vi "Teleop.vi"(10 "Match Info":T3={"Autonomous Elapsed Seconds"=0.0, "TeleOp Elapsed Seconds"=0.0, "Disabled Elapsed Seconds"=0.0, "Visited Autonomous"=FALSE, "Visited TeleOp"=FALSE, "Visited Disabled"=FALSE, "Autonomous Settings"={"Autonomous Style"=enum."Independent", "VI Refnum"=refnum}}, 11 "Call Context":T4) -> ()   [LabVIEW 2011]
doc: "This VI is called for each TeleOp packet received from the DS where the robot is not disabled. It is often used to read from the joysticks and update I/O or to update setpoints for timed control loops. It should complete and return within 20 milliseconds or it may miss DS packets."
uses:
  <vilib>/Rock Robotics/WPI/DriverStation/WPI_DriverStationDerivedRobotMode.ctl
  <vilib>/Rock Robotics/WPI/DriverStation/WPI_DriverStationMatch Info.ctl
  <vilib>/Rock Robotics/WPI/Relay/WPI_RelayValue.ctl
  Robot Global Data.vi
  <vilib>/addons/control/pid/pid.llb/PID (DBL).vi
  <vilib>/addons/control/pid/NI_PID_pid.lvlib
panel:
  in  "PID gains":T1={"proportional gain (Kc)"=0.0006, "integral time (Ti, min)"=0.03333, "derivative time (Td, min)"=0.002} {"derivative time (Td, min)" format="%.5f"; "integral time (Ti, min)" format="%.5f"; "proportional gain (Kc)" format="%.5f"}
  in  "PID Setpoint":dbl(knob) scale=0.0..2000.0
  in  "Light":bool
  in  "Drive Mode":T2(ring)=enum."Manual"
  in  "RPM Set Point 2":dbl(knob) scale=0.0..2000.0
  in  "RPM Gain (Edan Test)":dbl
  in  "Right Wheel Gain":dbl
  in  "Left Wheel Gain":dbl
  out "pythagorean X":dbl(knob) scale=0.0..20.0
  out "camera distance":dbl(knob) scale=0.0..10.0
  out "Angle (X)":dbl
  out "pythagorean Y":dbl(knob) scale=0.0..20.0
  out "Angle (Y)":dbl
  in  "Boolean":bool
  in  "RPM Set Point":dbl(knob) scale=0.0..2000.0
  in  "Shooter Speed Gain":dbl=0.1
  in  "Angle Set Point":dbl(knob)=195.27022900531597 scale=180.0..220.0
  in  "Angle Gain":dbl
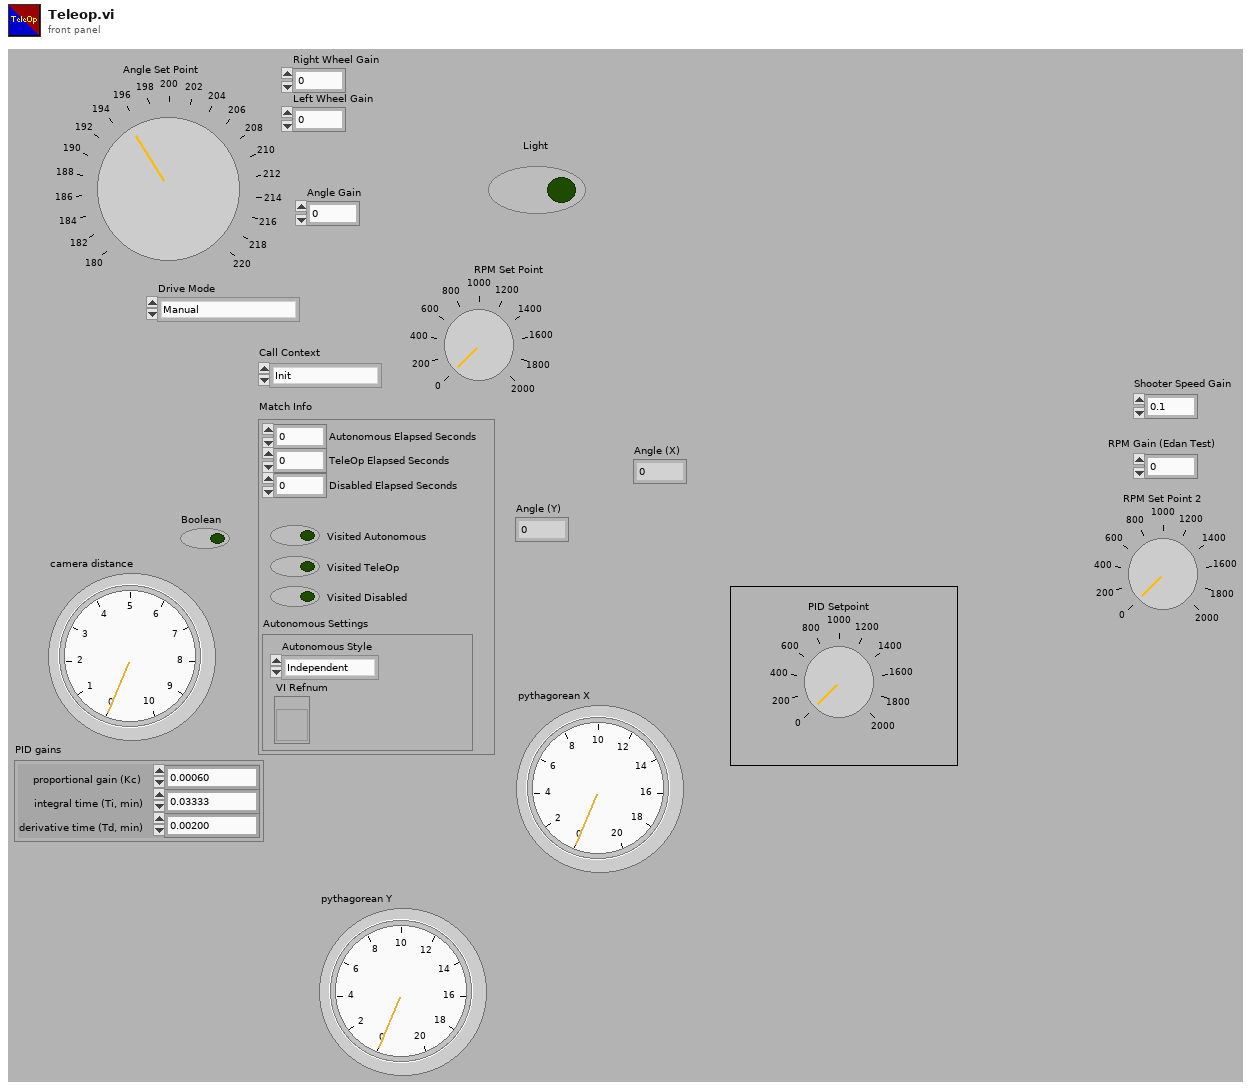
[diagram p1: front panel]
types:
  T1 = cluster{"proportional gain (Kc)":dbl, "integral time (Ti, min)":dbl, "derivative time (Td, min)":dbl}
  T2 = enum16{"Closed Loop Test", "PID Shooter Test", "camera", "ClosedLoopDrive", "Manual", "shooter test"}
  T3 = typedef "WPI_DriverStationMatch Info.ctl" = cluster{"Autonomous Elapsed Seconds":dbl, "TeleOp Elapsed Seconds":dbl, "Disabled Elapsed Seconds":dbl, "Visited Autonomous":bool, "Visited TeleOp":bool, "Visited Disabled":bool, "Autonomous Settings":cluster{"Autonomous Style":enum16{"Iterative", "Independent"}, "VI Refnum":refnum<vi>}}
  T4 = typedef "WPI_DriverStationDerivedRobotMode.ctl" = enum16{"Init", "Execute", "Stop"}
  T5 = typedef "WPI_RelayValue.ctl" = enum16{"Off", "On", "Forward", "Reverse"}
  T6 = typedef "WPI_MotorControlDeviceRef.ctl" = cluster{"DeviceStatus":errorcluster, "Type":enum16{"PWM", "CAN"}, "PWM":cluster{"Digital Module":T7, "PWM Channel":T8, "DeadBand":T9}, "CAN":cluster{"Device Number":u8, "Control Mode":T10, "Semaphore":T11, "Max Vout":dbl}, "Invert":bool, "TransformRef":T12, "InvTransformRef":T12}
  T7 = typedef "FPGA_TypedefDigitalModule.ctl" = enum16{"Digital Module 1", "Digital Module 2"}
  T8 = typedef "FPGA_DIOPWMChannel.ctl" = enum8{"PWM 1", "PWM 2", "PWM 3", "PWM 4", "PWM 5", "PWM 6", "PWM 7", "PWM 8", "PWM 9", "PWM 10", "Invalid"}
  T9 = typedef "WPI_PWMDeadband.ctl" = cluster{"Name":string, "maxPositivePwm":i32, "minPositivePwm":i32, "centerPwm":i32, "maxNegativePwm":i32, "minNegativePwm":i32, "angularRange":u16}
  T10 = typedef "WPI_CANJaguar_ControlMode.ctl" = enum8{"Percent VBus", "Current", "Speed", "Position", "Voltage"}
  T11 = typedef "Semaphore RefNum" = refnum<k1>
  T12 = typedef "WPI_PWMTransform_ConPane.ctl" = refnum<vi>
  T13 = typedef "WPI_DigitalInputDevRef.ctl" = cluster{"DevStatus":errorcluster, "DIO Channel":T14, "Digital Module":T7}
  T14 = typedef "FPGA_DIOChannel.ctl" = enum8{"DIO 1", "DIO 2", "DIO 3", "DIO 4", "DIO 5", "DIO 6", "DIO 7", "DIO 8", "DIO 9", "DIO 10", "DIO 11", "DIO 12", "DIO 13", "DIO 14", "Invalid"}
  T15 = typedef "WPI_JoystickDevRef.ctl" = cluster{"Device":T16}
  T16 = typedef "WPI_JoystickDeviceEnum.ctl" = enum16{"USB 1", "USB 2", "USB 3", "USB 4", "Kinect 1", "Kinect 2"}
  T17 = typedef "WPI_JoystickButtonState.ctl" = cluster{"Button 1":bool, "Button 2":bool, "Button 3":bool, "Button 4":bool, "Button 5":bool, "Button 6":bool, "Button 7":bool, "Button 8":bool, "Button 9":bool, "Button 10":bool, "Button 11":bool, "Button 12":bool}
  T18 = cluster{"axis 1 (x)":dbl, "axis 2 (y)":dbl, "axis 3 (throttle)":dbl, "axis 4":dbl, "axis 5":dbl, "axis 6":dbl}
  T19 = typedef "WPI_RelayDevRef.ctl" = cluster{"DevStatus":errorcluster, "Relay Channel":T20, "Digital Module":T7, "Relay Direction":T21}
  T20 = typedef "FPGA_DIORelayChannel.ctl" = enum8{"Relay 1", "Relay 2", "Relay 3", "Relay 4", "Relay 5", "Relay 6", "Relay 7", "Relay 8", "Invalid"}
  T21 = typedef "WPI_RelayDirection.ctl" = enum16{"Both directions", "Forward only", "Reverse only"}
  T22 = typedef "WPI_RobotDriveDevRef.ctl" = cluster{"DevStatus":errorcluster, "Motors[]":T6[], "Square Inputs":bool, "Max Output":dbl, "Isochronous":bool}
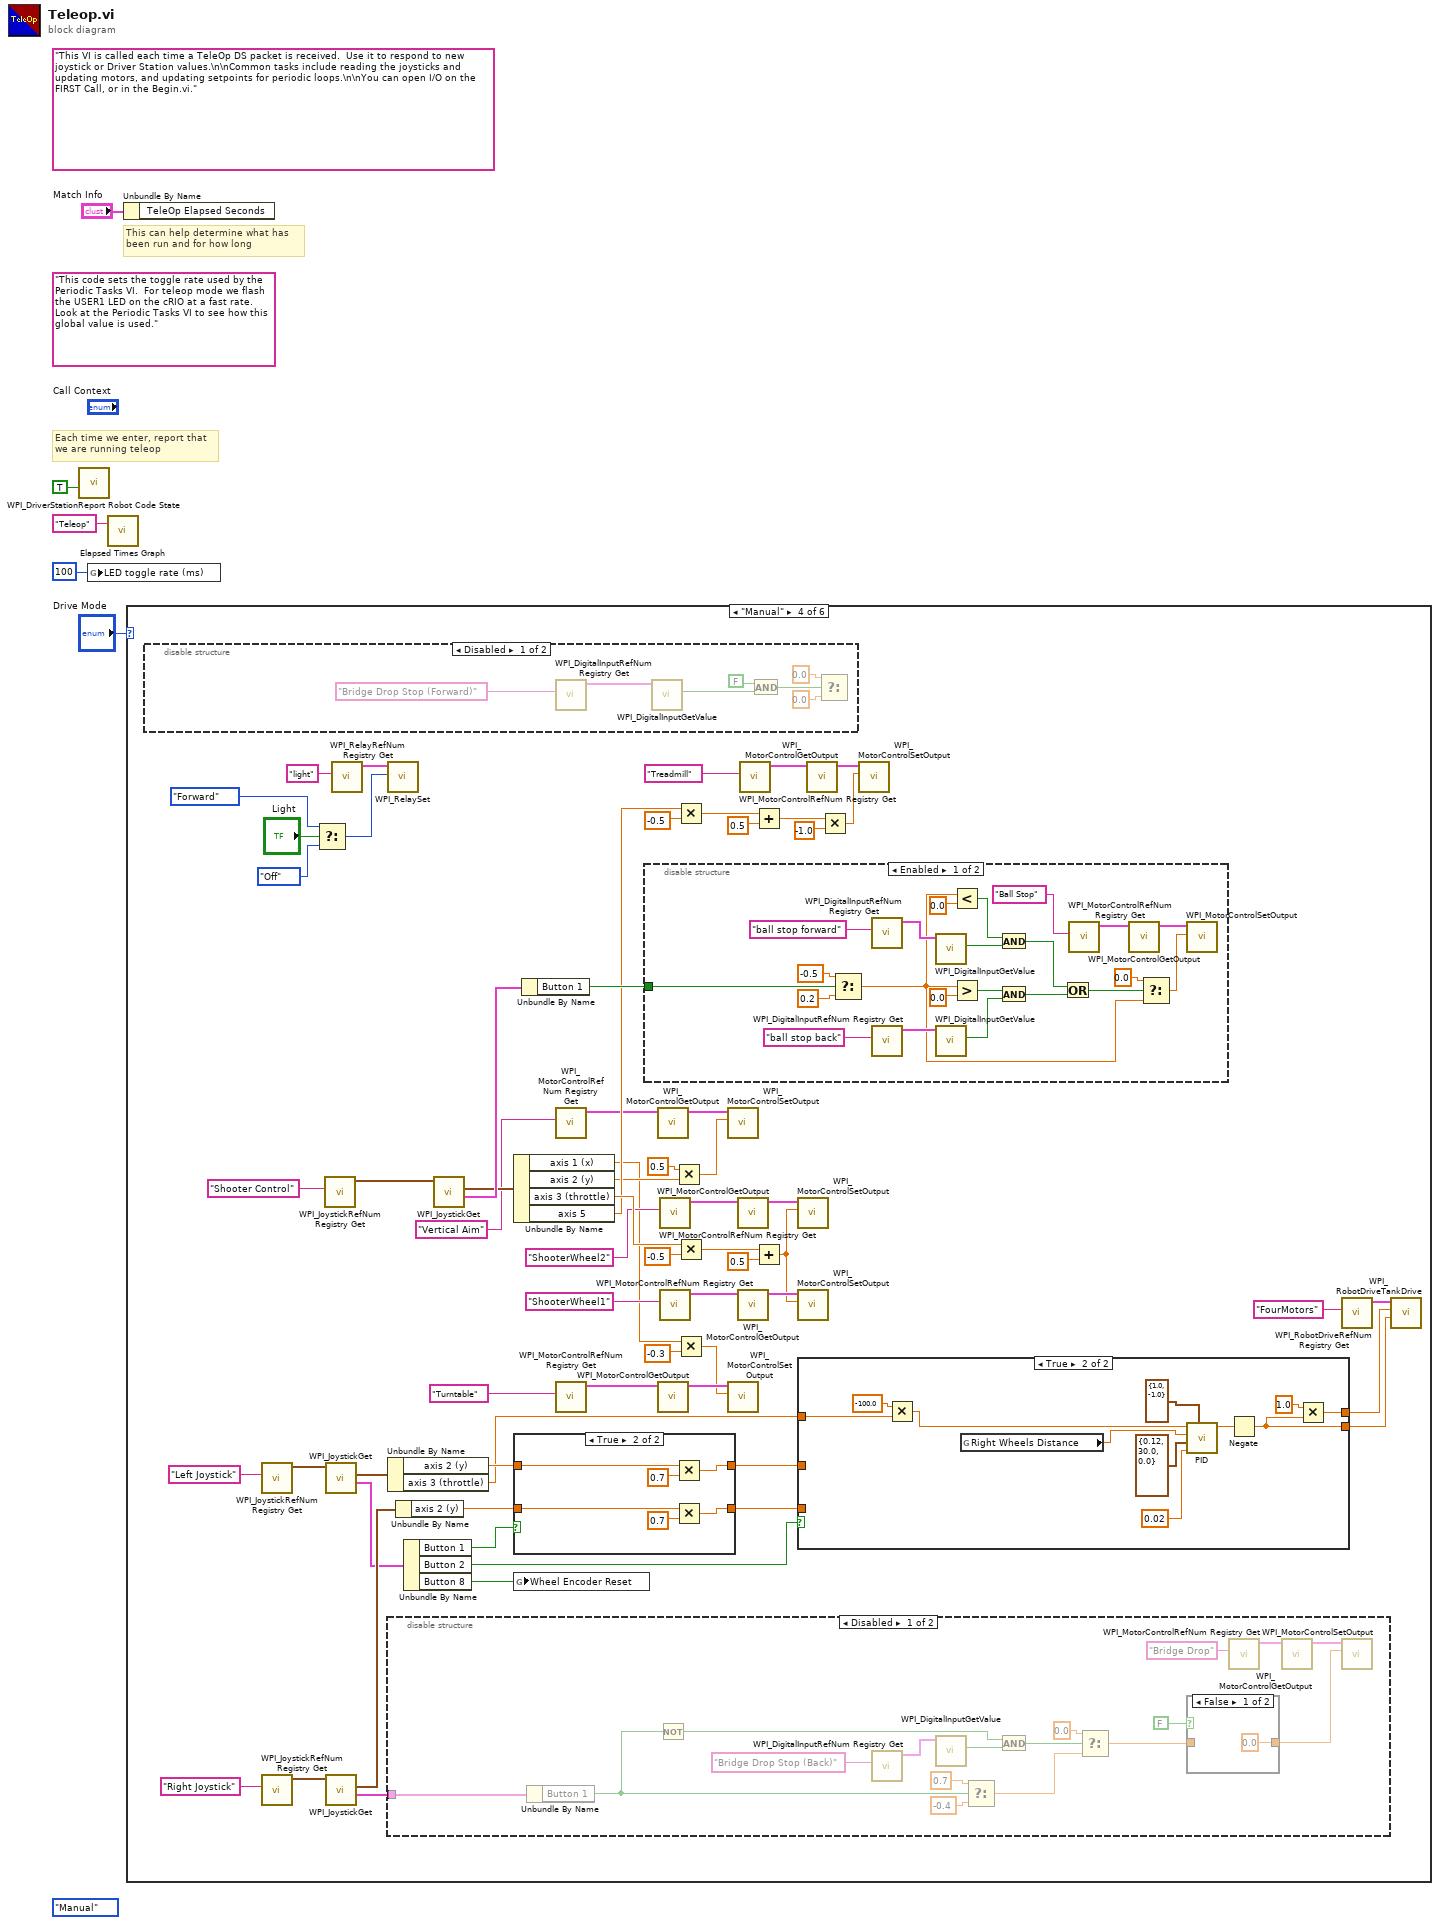
[diagram p0: block diagram]
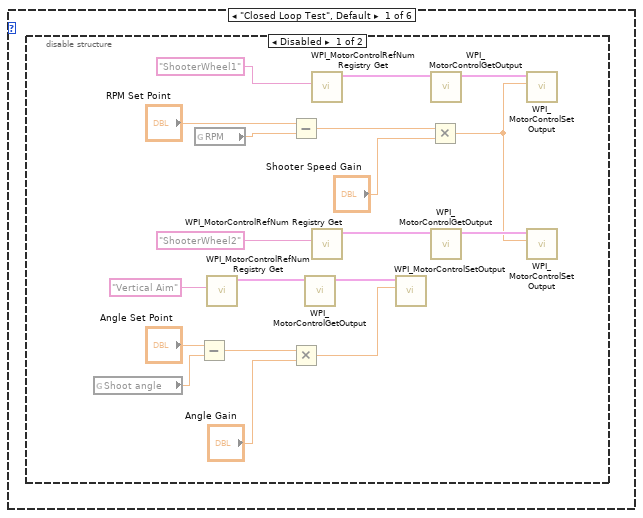
[diagram p2: hidden frame]
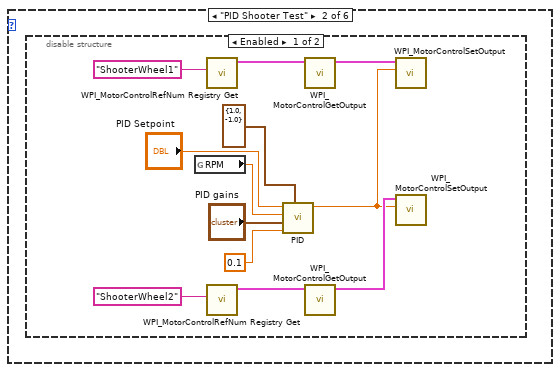
[diagram p4: hidden frame]
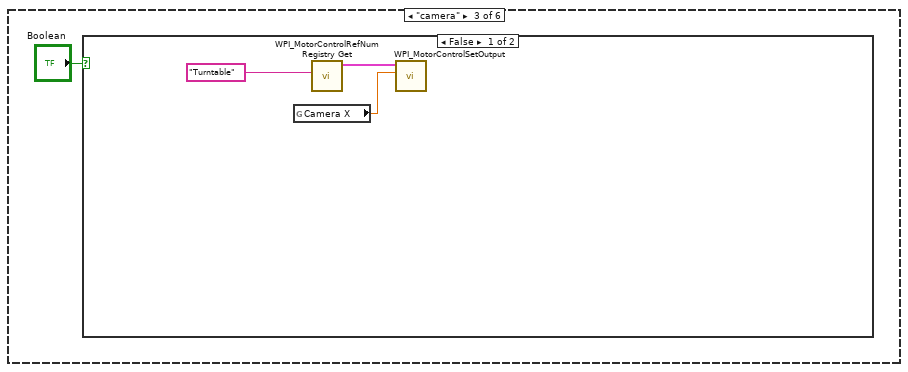
[diagram p6: hidden frame]
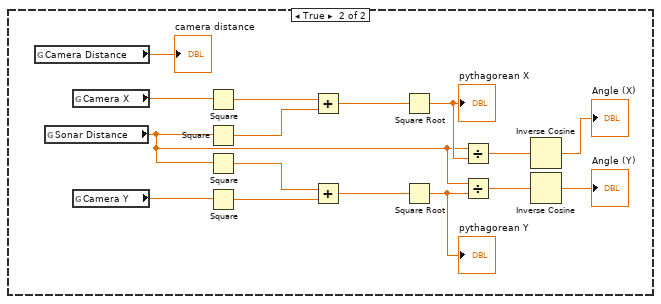
[diagram p7: hidden frame]
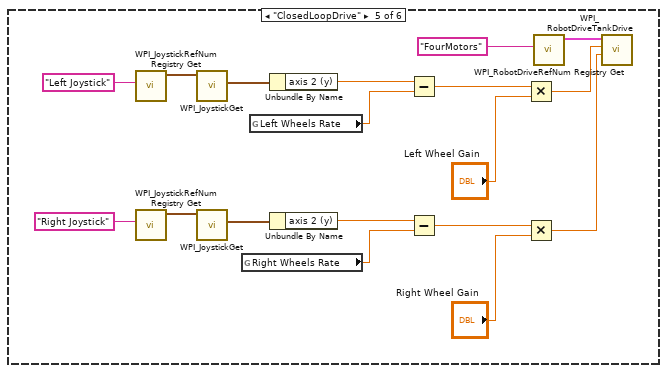
[diagram p14: hidden frame]
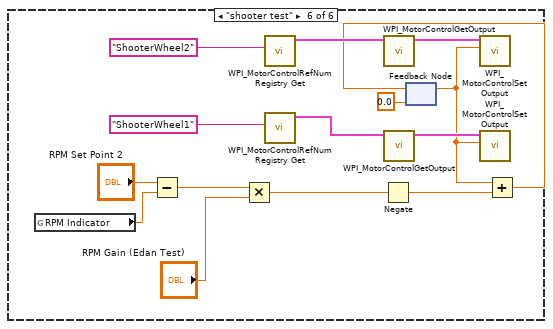
[diagram p15: hidden frame]
diagram:
  (unwired) T2."Manual" ("Drive Mode")
  (unwired) "This code sets the toggle rate used by the Periodic Tasks VI.  For teleop mode we flash the USER1 LED on the cRIO at a fast rate.  Look at the Periodic Tasks VI to see how this global value is used."
  (unwired) "This VI is called each time a TeleOp DS packet is received.  Use it to respond to new joystick or Driver Station values.\n\nCommon tasks include reading the joysticks and updating motors, and updating setpoints for periodic loops.\n\nYou can open I/O on the FIRST Call, or in the Begin.vi."
  # "Each time we enter, report that\nwe are running teleop"
  # "This can help determine what has\nbeen run and for how long"
  n1 = call <vilib>:"WPI_DriverStationReport Robot Code State.vi"("TeleOp"=TRUE ("Autonomous")) -> ()  [unwired: 10 in, 1 out]
  n2 = global write "Robot Global Data.vi" "LED toggle rate (ms)"(u32 100 ("LED ms toggle rate")) -> ()
  n3 = call "Elapsed Times Graph.vi"("User Identification:"="Teleop") -> ()  [unwired: 3 in]
  n4 = Unbundle By Name("Match Info") -> ()  [unwired: 1 out]
  n5 = case shown="\"Manual\"" "Drive Mode" {
    frame "Closed Loop Test", Default {
      n6 = disable-structure shown="Disabled" {
        frame Disabled {
          n7 = global read "Robot Global Data.vi" "Shoot angle"() -> (w14:dbl)
          n8 = global read "Robot Global Data.vi" "RPM"() -> (w18:dbl)
          n9 = Subtract(x="Angle Set Point", y=w14) -> (x-y=w12:dbl)
          n10 = call <vilib>:"WPI_MotorControlRefNum Registry Get.vi"("refnum name"="Vertical Aim") -> ("MotorControlDevRef"=w8:T6)  [unwired: 9 in, 1 out]
          n11 = Subtract(x="RPM Set Point", y=w18) -> (x-y=w16:dbl)
          n12 = Multiply(x=w12, y="Angle Gain") -> (x*y=w10:dbl)
          n13 = call <vilib>:"WPI_MotorControlGetOutput.vi"("MotorControlDevRef"=w8) -> ("MotorControlDevRef"=w9:T6)  [unwired: 8 in, 2 out]
          n14 = call <vilib>:"WPI_MotorControlRefNum Registry Get.vi"("refnum name"="ShooterWheel1") -> ("MotorControlDevRef"=w19:T6)  [unwired: 9 in, 1 out]
          n15 = call <vilib>:"WPI_MotorControlRefNum Registry Get.vi"("refnum name"="ShooterWheel2") -> ("MotorControlDevRef"=w23:T6)  [unwired: 9 in, 1 out]
          n16 = call <vilib>:"WPI_MotorControlSetOutput.vi"("Output"=w10, "MotorControlDevRef"=w9) -> ()  [unwired: 8 in, 2 out]
          n17 = Multiply(x=w16, y="Shooter Speed Gain") -> (x*y=w6:dbl)
          n18 = call <vilib>:"WPI_MotorControlGetOutput.vi"("MotorControlDevRef"=w19) -> ("MotorControlDevRef"=w20:T6)  [unwired: 8 in, 2 out]
          n19 = call <vilib>:"WPI_MotorControlGetOutput.vi"("MotorControlDevRef"=w23) -> ("MotorControlDevRef"=w22:T6)  [unwired: 8 in, 2 out]
          n20 = call <vilib>:"WPI_MotorControlSetOutput.vi"("Output"=w6, "MotorControlDevRef"=w20) -> ()  [unwired: 8 in, 2 out]
          n21 = call <vilib>:"WPI_MotorControlSetOutput.vi"("Output"=w6, "MotorControlDevRef"=w22) -> ()  [unwired: 8 in, 2 out]
        }
        frame Enabled {
        }
      }
    }
    frame "PID Shooter Test" {
      n22 = disable-structure shown="Enabled" {
        frame Enabled {
          n23 = global read "Robot Global Data.vi" "RPM"() -> (w30:dbl)
          n24 = call <vilib>:"WPI_MotorControlRefNum Registry Get.vi"("refnum name"="ShooterWheel1") -> ("MotorControlDevRef"=w31:T6)  [unwired: 9 in, 1 out]
          n25 = call <vilib>:"WPI_MotorControlRefNum Registry Get.vi"("refnum name"="ShooterWheel2") -> ("MotorControlDevRef"=w35:T6)  [unwired: 9 in, 1 out]
          n26 = call-poly <vilib>:"PID.vi"("output range"=cluster{"output high":dbl, "output low":dbl} {"output high"=1.0, "output low"=-1.0}, "dt (s)"=0.1, "PID gains"="PID gains", "process variable"=w30, "setpoint"="PID Setpoint") -> ("output"=w26:dbl)  [unwired: 5 in, 1 out]
          n27 = call <vilib>:"WPI_MotorControlGetOutput.vi"("MotorControlDevRef"=w31) -> ("MotorControlDevRef"=w32:T6)  [unwired: 8 in, 2 out]
          n28 = call <vilib>:"WPI_MotorControlGetOutput.vi"("MotorControlDevRef"=w35) -> ("MotorControlDevRef"=w34:T6)  [unwired: 8 in, 2 out]
          n29 = call <vilib>:"WPI_MotorControlSetOutput.vi"("Output"=w26, "MotorControlDevRef"=w32) -> ()  [unwired: 8 in, 2 out]
          n30 = call <vilib>:"WPI_MotorControlSetOutput.vi"("Output"=w26, "MotorControlDevRef"=w34) -> ()  [unwired: 8 in, 2 out]
        }
        frame Disabled {
        }
      }
    }
    frame "camera" {
      n31 = case shown="False" "Boolean" {
        frame False {
          n32 = global read "Robot Global Data.vi" "Camera X"() -> (w38:dbl)
          n33 = call <vilib>:"WPI_MotorControlRefNum Registry Get.vi"("refnum name"="Turntable") -> ("MotorControlDevRef"=w40:T6)  [unwired: 9 in, 1 out]
          n34 = call <vilib>:"WPI_MotorControlSetOutput.vi"("Output"=w38, "MotorControlDevRef"=w40) -> ()  [unwired: 8 in, 2 out]
        }
        frame True {
          n35 = global read "Robot Global Data.vi" "Camera Distance"() -> (→"camera distance":dbl)
          n36 = global read "Robot Global Data.vi" "Sonar Distance"() -> (w53:dbl)
          n37 = global read "Robot Global Data.vi" "Camera X"() -> (w55:dbl)
          n38 = global read "Robot Global Data.vi" "Camera Y"() -> (w49:dbl)
          n39 = Square(x=w55) -> (x^2=w42:dbl)
          n40 = Square(x=w53) -> (x^2=w41:dbl)
          n41 = Square(x=w53) -> (x^2=w46:dbl)
          n42 = Square(x=w49) -> (x^2=w47:dbl)
          n43 = Add(x=w42, y=w41) -> (x+y=w43:dbl)
          n44 = Add(x=w46, y=w47) -> (x+y=w48:dbl)
          n45 = Square Root(x=w43) -> (sqrt(x)=w54:dbl)
          "pythagorean X" <- w54
          n46 = Square Root(x=w48) -> (sqrt(x)=w52:dbl)
          "pythagorean Y" <- w52
          n47 = Divide(x=w53, y=w54) -> (x/y=w45:dbl)
          n48 = Divide(x=w53, y=w52) -> (x/y=w50:dbl)
          n49 = Inverse Cosine(1:w45) -> (0:→"Angle (X)":dbl)
          n50 = Inverse Cosine(1:w50) -> (0:→"Angle (Y)":dbl)
        }
      }
    }
    frame "Manual" {
      n51 = disable-structure shown="Disabled" {
        frame Disabled {
          n52 = call <vilib>:"WPI_DigitalInputRefNum Registry Get.vi"("refnum name"="Bridge Drop Stop (Forward)") -> ("DigitalInputDevRef"=w159:T13)  [unwired: 9 in, 1 out]
          n53 = call <vilib>:"WPI_DigitalInputGetValue.vi"("DigitalInputDevRef"=w159) -> ("Value"=w158:bool)  [unwired: 8 in, 2 out]
          n54 = And(x=FALSE, y=w158) -> (x .and. y?=w157:bool)
          n55 = Select(t=0.0, s=w157, f=0.0) -> ()  [unwired: 1 out]
        }
        frame Enabled {
        }
      }
      n56 = call <vilib>:"WPI_JoystickRefNum Registry Get.vi"("refnum name"="Left Joystick") -> ("JoystickDevRef"=w115:T15)  [unwired: 9 in, 1 out]
      n57 = call <vilib>:"WPI_JoystickRefNum Registry Get.vi"("refnum name"="Right Joystick") -> ("JoystickDevRef"=w118:T15)  [unwired: 9 in, 1 out]
      n58 = Select(t=WPI_RelayValue."Forward" ("RelayValue"), s="Light", f=WPI_RelayValue."Off" ("RelayValue")) -> (s? t:f=w71:T5)
      n59 = call <vilib>:"WPI_JoystickRefNum Registry Get.vi"("refnum name"="Shooter Control") -> ("JoystickDevRef"=w88:T15)  [unwired: 9 in, 1 out]
      n60 = call <vilib>:"WPI_JoystickGet.vi"("JoystickDevRef"=w115) -> ("Buttons"=w67:T17, "Axes"=w116:T18)  [unwired: 4 in, 1 out]
      n61 = call <vilib>:"WPI_JoystickGet.vi"("JoystickDevRef"=w118) -> ("Buttons"=w77:T17, "Axes"=w119:T18)  [unwired: 4 in, 1 out]
      n62 = call <vilib>:"WPI_RelayRefNum Registry Get.vi"("refnum name"="light") -> ("RelayDevRef"=w75:T19)  [unwired: 9 in, 1 out]
      n63 = call <vilib>:"WPI_RelaySet.vi"("RelayValue"=w71, "RelayDevRef"=w75) -> ()  [unwired: 8 in, 2 out]
      n64 = Unbundle By Name(w116) -> ("axis 2 (y)"=w69:dbl, "axis 3 (throttle)"=w58:dbl)
      n65 = disable-structure shown="Disabled" {
        disable-tunnel: w77 -> [w150 _]
        frame Disabled {
          n66 = Unbundle By Name(w150) -> ("Button 1"=w144:bool)
          n67 = Not(x=w144) -> (.not. x?=w145:bool)
          n68 = call <vilib>:"WPI_DigitalInputRefNum Registry Get.vi"("refnum name"="Bridge Drop Stop (Back)") -> ("DigitalInputDevRef"=w147:T13)  [unwired: 9 in, 1 out]
          n69 = call <vilib>:"WPI_DigitalInputGetValue.vi"("DigitalInputDevRef"=w147) -> ("Value"=w140:bool)  [unwired: 8 in, 2 out]
          n70 = Select(t=0.7, s=w144, f=-0.4) -> (s? t:f=w139:dbl)
          n71 = And(x=w145, y=w140) -> (x .and. y?=w146:bool)
          n72 = Select(t=0.0, s=w146, f=w139) -> (s? t:f=w141:dbl)
          n73 = case shown="False" FALSE {
            tunnel: [0.0 ("f") w152] -> w134
            tunnel: w141 -> [_ w152]
            frame False {
            }
            frame True {
            }
          }
          n74 = call <vilib>:"WPI_MotorControlRefNum Registry Get.vi"("refnum name"="Bridge Drop") -> ("MotorControlDevRef"=w138:T6)  [unwired: 9 in, 1 out]
          n75 = call <vilib>:"WPI_MotorControlGetOutput.vi"("MotorControlDevRef"=w138) -> ("MotorControlDevRef"=w137:T6)  [unwired: 8 in, 2 out]
          n76 = call <vilib>:"WPI_MotorControlSetOutput.vi"("Output"=w134, "MotorControlDevRef"=w137) -> ()  [unwired: 8 in, 2 out]
        }
        frame Enabled {
        }
      }
      n77 = Unbundle By Name(w119) -> ("axis 2 (y)"=w68:dbl)
      n78 = Unbundle By Name(w67) -> ("Button 1"=w66:bool, "Button 2"=w60:bool, "Button 8"=w57:bool)
      n79 = call <vilib>:"WPI_JoystickGet.vi"("JoystickDevRef"=w88) -> ("Buttons"=w111:T17, "Axes"=w90:T18)  [unwired: 4 in, 1 out]
      n80 = Unbundle By Name(w90) -> ("axis 1 (x)"=w78:dbl, "axis 2 (y)"=w83:dbl, "axis 3 (throttle)"=w110:dbl, "axis 5"=w109:dbl)
      n81 = case shown="True" w66 {
        tunnel: [w161 w167] -> w63
        tunnel: w69 -> [w161 w164]
        tunnel: [w160 w166] -> w61
        tunnel: w68 -> [w160 w165]
        frame False {
        }
        frame True {
          n82 = Multiply(x=w164, y=0.7) -> (x*y=w167:dbl)
          n83 = Multiply(x=w165, y=0.7) -> (x*y=w166:dbl)
        }
      }
      n84 = global write "Robot Global Data.vi" "Wheel Encoder Reset"(w57) -> ()
      n85 = Unbundle By Name(w111) -> ("Button 1"=w112:bool)
      n86 = call <vilib>:"WPI_MotorControlRefNum Registry Get.vi"("refnum name"="Vertical Aim") -> ("MotorControlDevRef"=w86:T6)  [unwired: 9 in, 1 out]
      n87 = call <vilib>:"WPI_MotorControlRefNum Registry Get.vi"("refnum name"="Turntable") -> ("MotorControlDevRef"=w107:T6)  [unwired: 9 in, 1 out]
      n88 = disable-structure shown="Enabled" {
        disable-tunnel: w112 -> [w187 _]
        frame Enabled {
          n89 = Select(t=-0.5, s=w187, f=0.2) -> (s? t:f=w174:dbl)
          n90 = call <vilib>:"WPI_DigitalInputRefNum Registry Get.vi"("refnum name"="ball stop forward") -> ("DigitalInputDevRef"=w180:T13)  [unwired: 9 in, 1 out]
          n91 = call <vilib>:"WPI_DigitalInputRefNum Registry Get.vi"("refnum name"="ball stop back") -> ("DigitalInputDevRef"=w179:T13)  [unwired: 9 in, 1 out]
          n92 = call <vilib>:"WPI_DigitalInputGetValue.vi"("DigitalInputDevRef"=w180) -> ("Value"=w169:bool)  [unwired: 8 in, 2 out]
          n93 = call <vilib>:"WPI_DigitalInputGetValue.vi"("DigitalInputDevRef"=w179) -> ("Value"=w168:bool)  [unwired: 8 in, 2 out]
          n94 = Less?(x=w174, y=0.0) -> (x < y?=w170:bool)
          n95 = Greater?(x=w174, y=0.0) -> (0:w171:bool)
          n96 = And(x=w170, y=w169) -> (x .and. y?=w183:bool)
          n97 = And(x=w171, y=w168) -> (x .and. y?=w182:bool)
          n98 = Or(x=w183, y=w182) -> (x .or. y?=w181:bool)
          n99 = call <vilib>:"WPI_MotorControlRefNum Registry Get.vi"("refnum name"="Ball Stop") -> ("MotorControlDevRef"=w172:T6)  [unwired: 9 in, 1 out]
          n100 = call <vilib>:"WPI_MotorControlGetOutput.vi"("MotorControlDevRef"=w172) -> ("MotorControlDevRef"=w176:T6)  [unwired: 8 in, 2 out]
          n101 = Select(t=0.0, s=w181, f=w174) -> (s? t:f=w175:dbl)
          n102 = call <vilib>:"WPI_MotorControlSetOutput.vi"("Output"=w175, "MotorControlDevRef"=w176) -> ()  [unwired: 8 in, 2 out]
        }
        frame Disabled {
        }
      }
      n103 = call <vilib>:"WPI_MotorControlGetOutput.vi"("MotorControlDevRef"=w86) -> ("MotorControlDevRef"=w82:T6)  [unwired: 8 in, 2 out]
      n104 = call <vilib>:"WPI_MotorControlGetOutput.vi"("MotorControlDevRef"=w107) -> ("MotorControlDevRef"=w106:T6)  [unwired: 8 in, 2 out]
      n105 = call <vilib>:"WPI_MotorControlRefNum Registry Get.vi"("refnum name"="ShooterWheel2") -> ("MotorControlDevRef"=w101:T6)  [unwired: 9 in, 1 out]
      n106 = call <vilib>:"WPI_MotorControlRefNum Registry Get.vi"("refnum name"="ShooterWheel1") -> ("MotorControlDevRef"=w97:T6)  [unwired: 9 in, 1 out]
      n107 = Multiply(x=0.5 ("y"), y=w83) -> (x*y=w84:dbl)
      n108 = Multiply(x=w109, y=-0.5) -> (x*y=w94:dbl)
      n109 = Multiply(x=w110, y=-0.5) -> (x*y=w104:dbl)
      n110 = Multiply(x=w78, y=-0.3) -> (x*y=w65:dbl)
      n111 = call <vilib>:"WPI_MotorControlSetOutput.vi"("Output"=w84, "MotorControlDevRef"=w82) -> ()  [unwired: 8 in, 2 out]
      n112 = call <vilib>:"WPI_MotorControlSetOutput.vi"("Output"=w65, "MotorControlDevRef"=w106) -> ()  [unwired: 8 in, 2 out]
      n113 = call <vilib>:"WPI_MotorControlGetOutput.vi"("MotorControlDevRef"=w101) -> ("MotorControlDevRef"=w100:T6)  [unwired: 8 in, 2 out]
      n114 = call <vilib>:"WPI_MotorControlGetOutput.vi"("MotorControlDevRef"=w97) -> ("MotorControlDevRef"=w98:T6)  [unwired: 8 in, 2 out]
      n115 = call <vilib>:"WPI_MotorControlRefNum Registry Get.vi"("refnum name"="Treadmill") -> ("MotorControlDevRef"=w92:T6)  [unwired: 9 in, 1 out]
      n116 = Add(x=w94, y=0.5) -> (x+y=w79:dbl)
      n117 = Add(x=w104, y=0.5) -> (x+y=w76:dbl)
      n118 = call <vilib>:"WPI_MotorControlSetOutput.vi"("Output"=w76, "MotorControlDevRef"=w100) -> ()  [unwired: 8 in, 2 out]
      n119 = call <vilib>:"WPI_MotorControlSetOutput.vi"("Output"=w76, "MotorControlDevRef"=w98) -> ()  [unwired: 8 in, 2 out]
      n120 = case shown="True" w60 {
        tunnel: [w122 w125] -> w59
        tunnel: w63 -> [w122 _]
        tunnel: [w121 w124] -> w62
        tunnel: w61 -> [w121 _]
        tunnel: w58 -> [_ w132]
        frame False {
        }
        frame True {
          n121 = Multiply(x=-100.0, y=w132) -> (x*y=w133:dbl)
          n122 = global read "Robot Global Data.vi" "Right Wheels Distance"() -> (w130:dbl)
          n123 = call-poly <vilib>:"PID.vi"("output range"=cluster{"output high":dbl, "output low":dbl} {"output high"=1.0, "output low"=-1.0}, "dt (s)"=0.02, "PID gains"=T1 {"proportional gain (Kc)"=0.12, "integral time (Ti, min)"=30.0, "derivative time (Td, min)"=0.0}, "process variable"=w130, "setpoint"=w133) -> ("output"=w126:dbl)  [unwired: 5 in, 1 out]
          n124 = Negate(x=w126) -> (-x=w124:dbl)
          n125 = Multiply(x=1.0, y=w124) -> (x*y=w125:dbl)
        }
      }
      n126 = call <vilib>:"WPI_MotorControlGetOutput.vi"("MotorControlDevRef"=w92) -> ("MotorControlDevRef"=w91:T6)  [unwired: 8 in, 2 out]
      n127 = Multiply(x=w79, y=-1.0) -> (x*y=w80:dbl)
      n128 = call <vilib>:"WPI_MotorControlSetOutput.vi"("Output"=w80, "MotorControlDevRef"=w91) -> ()  [unwired: 8 in, 2 out]
      n129 = call <vilib>:"WPI_RobotDriveRefNum Registry Get.vi"("refnum name"="FourMotors") -> ("RobotDriveDevRef"=w114:T22)  [unwired: 1 in, 9 out]
      n130 = call <vilib>:"WPI_RobotDriveTankDrive.vi"("Right axis value"=w62, "Left axis value"=w59, "RobotDriveDevRef"=w114) -> ()  [unwired: 7 in, 2 out]
    }
    frame "ClosedLoopDrive" {
      n131 = call <vilib>:"WPI_JoystickRefNum Registry Get.vi"("refnum name"="Left Joystick") -> ("JoystickDevRef"=w202:T15)  [unwired: 9 in, 1 out]
      n132 = call <vilib>:"WPI_JoystickRefNum Registry Get.vi"("refnum name"="Right Joystick") -> ("JoystickDevRef"=w205:T15)  [unwired: 9 in, 1 out]
      n133 = call <vilib>:"WPI_JoystickGet.vi"("JoystickDevRef"=w202) -> ("Axes"=w203:T18)  [unwired: 4 in, 2 out]
      n134 = call <vilib>:"WPI_JoystickGet.vi"("JoystickDevRef"=w205) -> ("Axes"=w206:T18)  [unwired: 4 in, 2 out]
      n135 = global read "Robot Global Data.vi" "Right Wheels Rate"() -> (w198:dbl)
      n136 = global read "Robot Global Data.vi" "Left Wheels Rate"() -> (w196:dbl)
      n137 = Unbundle By Name(w203) -> ("axis 2 (y)"=w197:dbl)
      n138 = Unbundle By Name(w206) -> ("axis 2 (y)"=w199:dbl)
      n139 = Subtract(x=w197, y=w196) -> (x-y=w195:dbl)
      n140 = Subtract(x=w199, y=w198) -> (x-y=w193:dbl)
      n141 = Multiply(x=w195, y="Left Wheel Gain") -> (x*y=w194:dbl)
      n142 = Multiply(x=w193, y="Right Wheel Gain") -> (x*y=w192:dbl)
      n143 = call <vilib>:"WPI_RobotDriveRefNum Registry Get.vi"("refnum name"="FourMotors") -> ("RobotDriveDevRef"=w201:T22)  [unwired: 1 in, 9 out]
      n144 = call <vilib>:"WPI_RobotDriveTankDrive.vi"("Right axis value"=w192, "Left axis value"=w194, "RobotDriveDevRef"=w201) -> ()  [unwired: 7 in, 2 out]
    }
    frame "shooter test" {
      n145 = global read "Robot Global Data.vi" "RPM Indicator"() -> (w220:dbl)
      n146 = Subtract(x="RPM Set Point 2", y=w220) -> (x-y=w222:dbl)
      n147 = Multiply(x=w222, y="RPM Gain (Edan Test)") -> (x*y=w213:dbl)
      n148 = call <vilib>:"WPI_MotorControlRefNum Registry Get.vi"("refnum name"="ShooterWheel2") -> ("MotorControlDevRef"=w215:T6)  [unwired: 9 in, 1 out]
      n149 = call <vilib>:"WPI_MotorControlRefNum Registry Get.vi"("refnum name"="ShooterWheel1") -> ("MotorControlDevRef"=w219:T6)  [unwired: 9 in, 1 out]
      n150 = Negate(x=w213) -> (-x=w212:dbl)
      n151 = call <vilib>:"WPI_MotorControlGetOutput.vi"("MotorControlDevRef"=w215) -> ("MotorControlDevRef"=w216:T6)  [unwired: 8 in, 2 out]
      n152 = call <vilib>:"WPI_MotorControlGetOutput.vi"("MotorControlDevRef"=w219) -> ("MotorControlDevRef"=w218:T6)  [unwired: 8 in, 2 out]
      n153 = feedback #1(0.0) -> (w210:dbl)
      n154 = call <vilib>:"WPI_MotorControlSetOutput.vi"("Output"=w210, "MotorControlDevRef"=w216) -> ()  [unwired: 8 in, 2 out]
      n155 = call <vilib>:"WPI_MotorControlSetOutput.vi"("Output"=w210, "MotorControlDevRef"=w218) -> ()  [unwired: 8 in, 2 out]
      n156 = Add(x=w210, y=w212) -> (x+y=w211:dbl)
      n157 = feedback-in #1(w211) -> ()
    }
  }
